vi "CLD 10 Step Sequencer with CSV Front Panel.vi"() -> ()   [LabVIEW 2020]
doc: "CLD 10 Exercise"
panel:
  out "Step 3":bool
  out "Step 2":bool
  out "Step 1":bool
  out "Current Step time":dbl
  out "Time Has Elapsed":bool
  out "Elapsed Time (s)":string
  in  "Auto Reset":bool=TRUE
  in  "Reset Button":bool
  in  "Stop VI":bool
  out "error out":errorcluster
  in  "error in (no error)":errorcluster
  in  "Time Target (s)":dbl
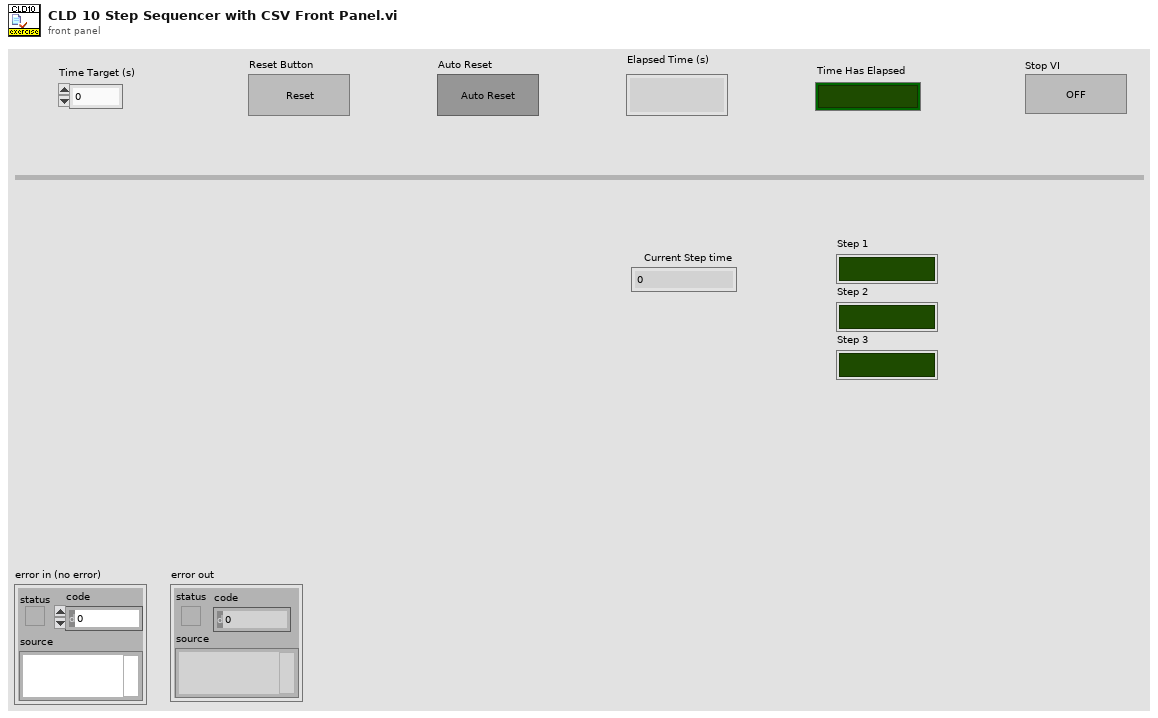
[diagram p1: front panel]
types:
  T1 = typedef "CLD 10 CSV file data structure.ctl" = cluster{"Step Time Target":i32, "Step 1":bool, "Step 2":bool, "Step 3":bool}
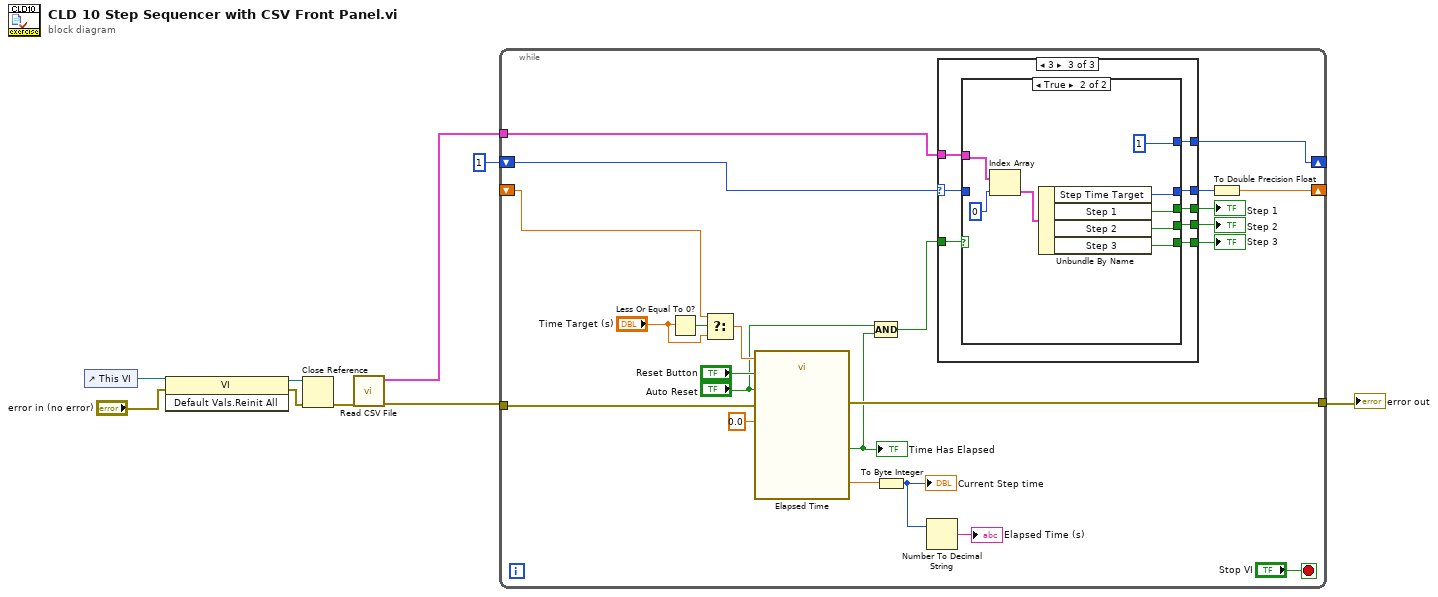
[diagram p0: block diagram]
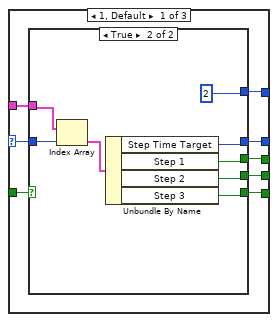
[diagram p2: hidden frame]
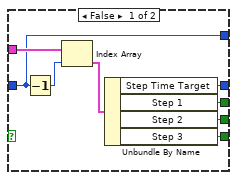
[diagram p3: hidden frame]
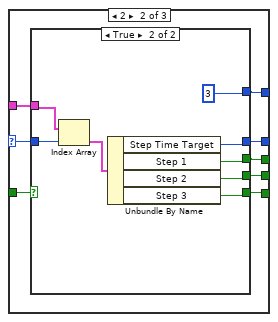
[diagram p4: hidden frame]
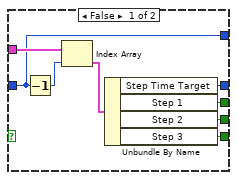
[diagram p5: hidden frame]
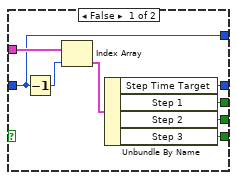
[diagram p6: hidden frame]
diagram:
  n1 = control-ref of="This VI"() -> (w7:refnum<vi>)
  n2 = invoke class="VI" method="Default Vals.Reinit All"(reference=w7, error in="error in (no error)") -> (reference out=w5:refnum<vi>, error out=w4:errorcluster)  [unwired: 1 in, 1 out]
  n3 = Close Reference(reference=w5, error in (no error)=w4) -> (error out=w3:errorcluster)
  n4 = call "Read CSV File.vi"("error in"=w3) -> ("error out"=w1:errorcluster, "Array"=w2:T1[])  [unwired: 9 in]
  n5 = while {
    tunnel: w1 -> [w31]
    shift-right: [w11] -> _
    shift-left: 1 -> [w10]
    tunnel: [w26] -> w8
    tunnel: w2 -> [w17]
    shift-right: [w19] -> _
    shift-left: _ -> [w18]
    stop <- "Stop VI" stop-if-true
    n6 = Less Or Equal To 0?(x="Time Target (s)") -> (x <= 0?=w30:bool)
    n7 = Select(t=w18, s=w30, f="Time Target (s)") -> (s? t:f=w28:dbl)
    n8 = call "Elapsed Time"("Time Target (s)"=w28, "Reset"="Reset Button", "Auto Reset"="Auto Reset", "error in (no error)"=w31, "Set Start Time (s)"=0.0) -> ("Elapsed Time (s)"=w22:dbl, "Time has Elapsed"=w24:bool, "error out"=w26:errorcluster)  [unwired: 7 in, 5 out]
    "Time Has Elapsed" <- w24
    n9 = Compound Arithmetic op=AND("Auto Reset", w24) -> (w12:bool)
    n10 = To Byte Integer(number=w22) -> (8bit integer=w21:i8)
    "Current Step time" <- w21
    n11 = Number To Decimal String(number=w21) -> (decimal integer string=→"Elapsed Time (s)":string)  [unwired: 1 in]
    n12 = case shown="3" w10 {
      selector: w10 -> [w39 w57 w87]
      tunnel: w17 -> [w40 w64 w88]
      tunnel: [w34 w63 w84] -> w16
      tunnel: [w37 w62 w83] -> w15
      tunnel: [w36 w61 w82] -> w14
      tunnel: [w35 w60 w81] -> w13
      tunnel: w12 -> [w38 w59 w86]
      tunnel: [w33 w58 w85] -> w11
      frame 1, Default {
        n13 = case shown="True" w38 {
          tunnel: w40 -> [w48 w55]
          tunnel: w39 -> [w41 w50]
          tunnel: [w45 w54] -> w34
          tunnel: [w44 w53] -> w37
          tunnel: [w43 w52] -> w36
          tunnel: [w42 w51] -> w35
          tunnel: [w41 2] -> w33
          frame False {
            n14 = Decrement(x=w41) -> (x-1=w47:i32)
            n15 = Index Array(array=w48, index=w47) -> (element=w46:T1)
            n16 = Unbundle By Name(w46) -> ("Step Time Target"=w45:i32, "Step 1"=w44:bool, "Step 2"=w43:bool, "Step 3"=w42:bool)
          }
          frame True {
            n17 = Index Array(array=w55, index=w50) -> (element=w56:T1)
            n18 = Unbundle By Name(w56) -> ("Step Time Target"=w54:i32, "Step 1"=w53:bool, "Step 2"=w52:bool, "Step 3"=w51:bool)
          }
        }
      }
      frame 2 {
        n19 = case shown="True" w59 {
          tunnel: w64 -> [w72 w79]
          tunnel: w57 -> [w65 w74]
          tunnel: [w69 w78] -> w63
          tunnel: [w68 w77] -> w62
          tunnel: [w67 w76] -> w61
          tunnel: [w66 w75] -> w60
          tunnel: [w65 3] -> w58
          frame False {
            n20 = Decrement(x=w65) -> (x-1=w71:i32)
            n21 = Index Array(array=w72, index=w71) -> (element=w70:T1)
            n22 = Unbundle By Name(w70) -> ("Step Time Target"=w69:i32, "Step 1"=w68:bool, "Step 2"=w67:bool, "Step 3"=w66:bool)
          }
          frame True {
            n23 = Index Array(array=w79, index=w74) -> (element=w80:T1)
            n24 = Unbundle By Name(w80) -> ("Step Time Target"=w78:i32, "Step 1"=w77:bool, "Step 2"=w76:bool, "Step 3"=w75:bool)
          }
        }
      }
      frame 3 {
        n25 = case shown="True" w86 {
          tunnel: w88 -> [w96 w103]
          tunnel: w87 -> [w89 _]
          tunnel: [w93 w102] -> w84
          tunnel: [w92 w101] -> w83
          tunnel: [w91 w100] -> w82
          tunnel: [w90 w99] -> w81
          tunnel: [w89 1] -> w85
          frame False {
            n26 = Decrement(x=w89) -> (x-1=w95:i32)
            n27 = Index Array(array=w96, index=w95) -> (element=w94:T1)
            n28 = Unbundle By Name(w94) -> ("Step Time Target"=w93:i32, "Step 1"=w92:bool, "Step 2"=w91:bool, "Step 3"=w90:bool)
          }
          frame True {
            n29 = Index Array(array=w103, index=0) -> (element=w104:T1)
            n30 = Unbundle By Name(w104) -> ("Step Time Target"=w102:i32, "Step 1"=w101:bool, "Step 2"=w100:bool, "Step 3"=w99:bool)
          }
        }
      }
    }
    "Step 1" <- w15
    "Step 2" <- w14
    "Step 3" <- w13
    n31 = To Double Precision Float(number=w16) -> (double precision float=w19:dbl)
  }
  "error out" <- w8
